vi "Path Array to Path String.vi"(11 "path array":string[](array[string])) -> (3 "path":string)   [LabVIEW 2017, in "Variant Data Manipulation.lvlib"]
uses:
  Variant Data Manipulation.lvlib
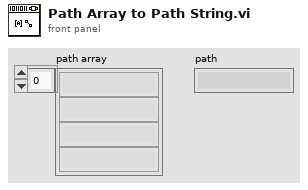
[diagram p1: front panel]
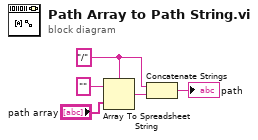
[diagram p0: block diagram]
diagram:
  w2 = "/" ("delimiter (Tab)")
  n1 = Array To Spreadsheet String(delimiter (Tab)=w2, array="path array", 3:"" ("format string")) -> (spreadsheet string=w1:string)
  n2 = Concatenate Strings(w2, w1) -> (→"path":string)
